vi "Hall Effect Calculations.vi"(0 "Thickness (cm)":dbl, 1 "Hall Voltage Array":dbl[](array[numeric]), 5 "Current (A)":dbl, 7 "pAVG":dbl, 9 "Flux":dbl, 11 "error":errorcluster) -> (4 "RHAVG":dbl, 6 "RHC":dbl, 8 "RHD":dbl, 10 "Hall Mobility":dbl, 14 "n/p":dbl, 15 "error out":errorcluster)   [LabVIEW 2016, in "Hall Effect Library.lvlib"]
uses:
  Hall Effect Library.lvlib
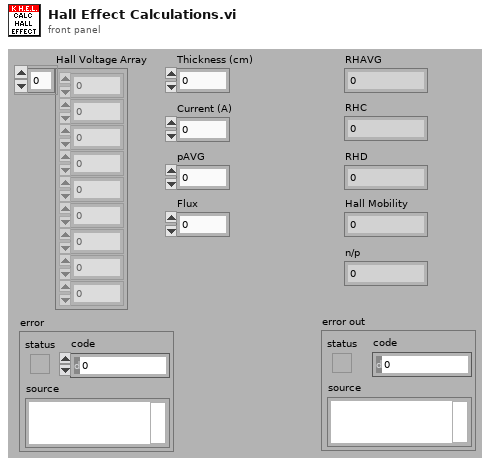
[diagram p1: front panel]
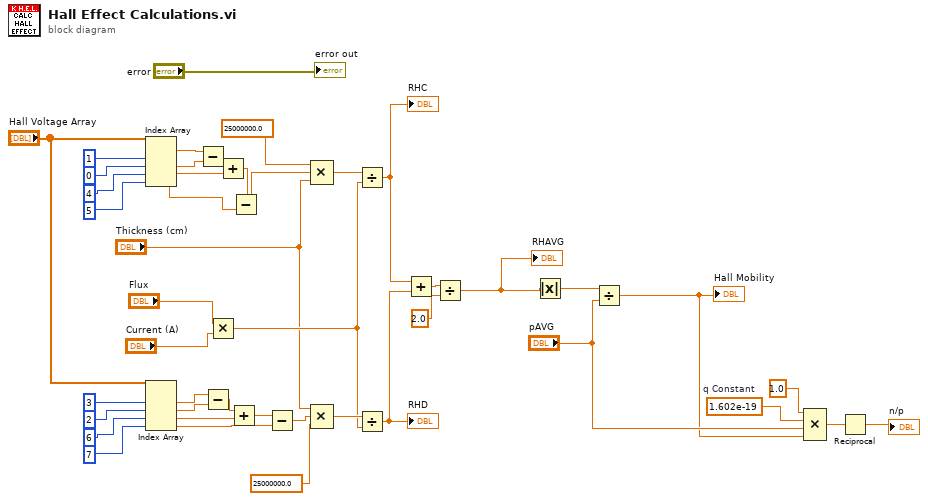
[diagram p0: block diagram]
diagram:
  w9 = 1.602e-19  # q Constant
  n1 = Index Array(array="Hall Voltage Array", index #1=1 ("index"), index #2=0 ("index"), index #3=4 ("index"), index #4=5 ("index")) -> (element #1=w42:dbl, element #2=w41:dbl, element #3=w21:dbl, element #4=w19:dbl)
  n2 = Index Array(array="Hall Voltage Array", index #1=3 ("index"), index #2=2 ("index"), index #3=6 ("index"), index #4=7 ("index")) -> (element #1=w30:dbl, element #2=w31:dbl, element #3=w16:dbl, element #4=w15:dbl)
  n3 = Subtract(x=w42, y=w41) -> (x-y=w40:dbl)
  n4 = Subtract(x=w30, y=w31) -> (x-y=w17:dbl)
  n5 = Multiply(x="Flux", y="Current (A)") -> (x*y=w6:dbl)
  n6 = Add(x=w40, y=w21) -> (x+y=w20:dbl)
  n7 = Add(x=w17, y=w16) -> (x+y=w14:dbl)
  n8 = Subtract(x=w20, y=w19) -> (x-y=w18:dbl)
  n9 = Subtract(x=w14, y=w15) -> (x-y=w13:dbl)
  n10 = Compound Arithmetic op=MULTIPLY(25000000.0 ("value"), w18, "Thickness (cm)") -> (w36:dbl)
  n11 = Compound Arithmetic op=MULTIPLY("Thickness (cm)", w13, 25000000.0 ("value")) -> (w25:dbl)
  n12 = Divide(x=w36, y=w6) -> (x/y=w8:dbl)
  "RHC" <- w8
  n13 = Divide(x=w25, y=w6) -> (x/y=w7:dbl)
  "RHD" <- w7
  n14 = Add(x=w8, y=w7) -> (x+y=w23:dbl)
  n15 = Divide(x=w23, y=2.0) -> (x/y=w2:dbl)
  "RHAVG" <- w2
  n16 = Absolute Value(x=w2) -> (abs(x)=w1:dbl)
  n17 = Divide(x=w1, y="pAVG") -> (x/y=w10:dbl)
  "Hall Mobility" <- w10
  n18 = Compound Arithmetic op=MULTIPLY(1.0 ("value"), w9, "pAVG", w10) -> (w12:dbl)
  n19 = Reciprocal(x=w12) -> (1/x=→"n/p":dbl)
  "error out" <- "error"
